vi "PriceData Randomize Demand.vi"(10 "DeviceID":T2) -> (3 "PriceData_Demand Array out":T1[](array[typedef]))   [LabVIEW 2018, in "IED Test Framework.lvlib" / "IED Test.lvclass"]
uses:
  IED Test.lvclass
  <vilib>/ORNL/CSEISMIC DDS/CSEISMIC DDS Base/Data Types/Controls/DeviceID.ctl
  <vilib>/ORNL/CSEISMIC DDS/CSEISMIC DDS Base/Data Types/PriceData_Demand.ctl
  <vilib>/ORNL/CSEISMIC DDS/CSEISMIC DDS Base/CSEISMIC DDS.lvclass
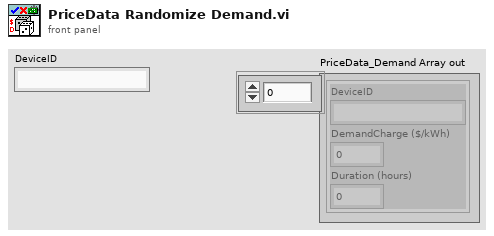
[diagram p1: front panel]
types:
  T1 = typedef "CSEISMIC DDS.lvlib/CSEISMIC DDS.lvclass/PriceData_Demand.ctl" = cluster{"DeviceID":T2, "DemandCharge ($/kWh)":dbl, "Duration (hours)":dbl}
  T2 = typedef "CSEISMIC DDS.lvlib/CSEISMIC DDS.lvclass/DeviceID.ctl" = string
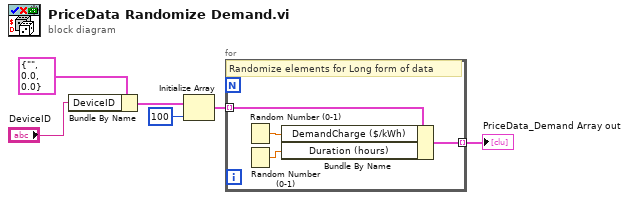
[diagram p0: block diagram]
diagram:
  n1 = Bundle By Name(cluster=T1 {"DeviceID"="", "DemandCharge ($/kWh)"=0.0, "Duration (hours)"=0.0} ("PriceData_Demand"), "DeviceID"="DeviceID") -> (w6:T1)
  n2 = Initialize Array(w6, 100 ("dimension size")) -> (w3:T1[])
  n3 = for {
    tunnel: w3 -> [w10] mode=indexing
    tunnel: [w9] -> w1 mode=indexing
    # "Randomize elements for Long form of data"
    n4 = Random Number (0-1)() -> (number: 0 to 1=w7:dbl)
    n5 = Random Number (0-1)() -> (number: 0 to 1=w8:dbl)
    n6 = Bundle By Name(cluster=w10, "DemandCharge ($/kWh)"=w7, "Duration (hours)"=w8) -> (w9:T1)
  }
  "PriceData_Demand Array out" <- w1
